vi "update destination folder.vi"(8 "error in":errorcluster, 11 "File in":refnum<class "File.lvclass">) -> (0 "error out":errorcluster, 3 "File out":refnum<class "File.lvclass">)   [LabVIEW 2023, in "File Classes.lvlib" / "File.lvclass"]
uses:
  File.lvclass
  File.lvclass/File.ctl
  File Classes.lvlib
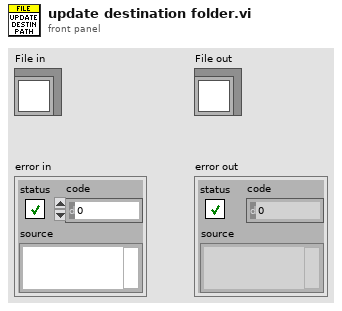
[diagram p1: front panel]
types:
  T1 = typedef "File Classes.lvlib/file operation settings mode.ctl" = enum16{"Copy Files", "Move Files", "Rename Files"}
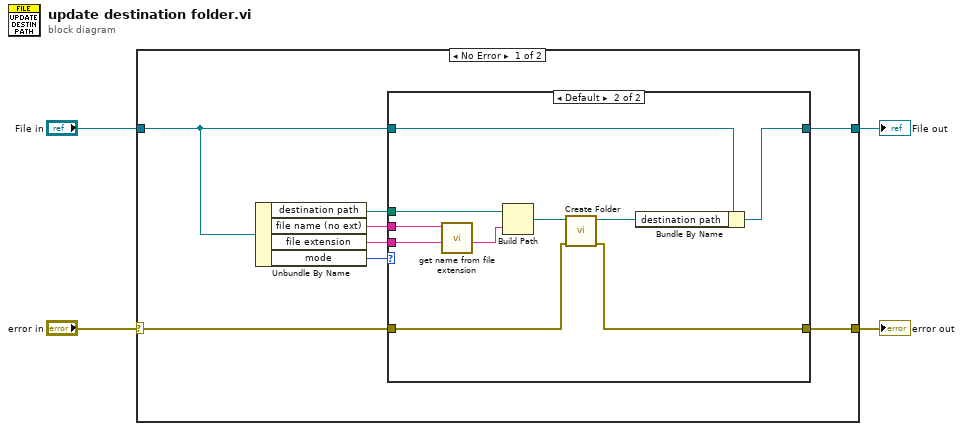
[diagram p0: block diagram]
diagram:
  n1 = case shown="No Error" "error in" {
    selector: "error in" -> [w9 w26]
    tunnel: [w8 w26] -> w3
    tunnel: [w12 w25] -> w1
    tunnel: "File in" -> [w11 w25]
    frame No Error {
      n2 = Unbundle By Name(w11) -> ("destination path"=w10:path, "file name (no ext)"=w7:string, "file extension"=w6:string, "mode"=w5:T1)
      n3 = case shown="Default" w5 {
        tunnel: [w14 w24] -> w12
        tunnel: w11 -> [w14 w23]
        tunnel: w10 -> [_ w22]
        tunnel: w9 -> [w13 w19]
        tunnel: [w13 w18] -> w8
        tunnel: w7 -> [_ w17]
        tunnel: w6 -> [_ w16]
        frame "Rename Files" {
        }
        frame Default {
          n4 = call "get name from file extension.vi"("file ext"=w16, "file name (no ext)"=w17) -> ("extension folder"=w20:string)  [unwired: 8 in, 1 out]
          n5 = Build Path(base path=w22, name or relative path=w20) -> (appended path=w21:path)
          n6 = call <userlib>:"Create Folder.vi"("error in"=w19, "Directory Path"=w21) -> ("error out"=w18:errorcluster, "dup Directory Path"=w15:path)  [unwired: 8 in]
          n7 = Bundle By Name(cluster=w23, "destination path"=w15) -> (w24:refnum<class "File.lvclass">)
        }
      }
    }
    frame Error {
    }
  }
  "error out" <- w3
  "File out" <- w1
